vi "set Defaults.vi"(0 "Session in":refnum<class "Snapshot.lvclass">, 11 "error in":errorcluster) -> (4 "Session out":refnum<class "Snapshot.lvclass">, 15 "error out":errorcluster)   [LabVIEW 2015, in "Snapshot.lvclass"]
uses:
  Snapshot.lvclass
  <userlib>/_Session Fwk/Session - Root.lvclass
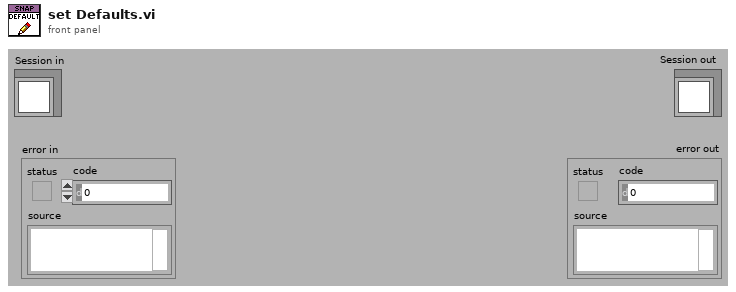
[diagram p1: front panel]
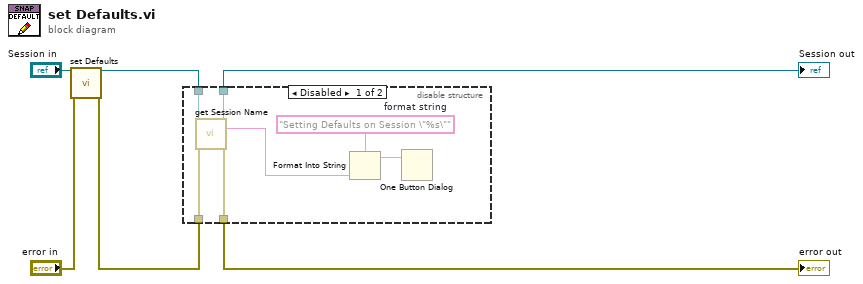
[diagram p0: block diagram]
diagram:
  n1 = call-parent "set Defaults.vi"("OBJ - Session in"="Session in", "error in"="error in") -> ("OBJ - Session out"=w3:refnum<class "Snapshot.lvclass">, "error out"=w1:errorcluster)  [unwired: 12 in]
  n2 = disable-structure shown="Disabled" {
    disable-tunnel: w3 -> [w13 w15]
    disable-tunnel: [w12 w15] -> w5
    disable-tunnel: w1 -> [w8 w14]
    disable-tunnel: [w7 w14] -> w6
    frame Disabled {
      w10 = "Setting Defaults on Session \"%s\""  # format string
      n3 = call <userlib>:"get Session Name.vi"("OBJ - Session in"=w13, "error in (no error)"=w8) -> ("OBJ - Session out"=w12:refnum<class "Snapshot.lvclass">, "Session Name"=w11:string, "error out"=w7:errorcluster)  [unwired: 11 in]
      n4 = Format Into String(format string=w10, w11) -> (resulting string=w9:string)  [unwired: 2 in, 1 out]
      n5 = One Button Dialog(message=w9) -> ()  [unwired: 1 in, 1 out]
    }
    frame Enabled {
    }
  }
  "error out" <- w6
  "Session out" <- w5
